vi "Insight_RW_Sweep_Power.vi"(7 "Parameter Type":enum16{"Value", "MAXimum", "MINimum", "DEFault"}(ring), 8 "error in (no error)":errorcluster, 9 "Mode (Read / Write)":enum8{"Write", "Read"}(ring), 10 "Power (mW)":dbl=5.0, 11 "telnet connection":T1) -> (0 "error out":errorcluster, 1 "response data":string, 2 "Power (mW)":dbl format="%.3g", 3 "telnet  connection out":T1)   [LabVIEW 2011]
doc: "Insight Photonic Solutions\n\nThis VI reads or writes the average power of the laser during a sweep.\n\nINPUTS\n\nMode - Tells the VI whether the command is a Read or a Write. (Default = Read).\nParameter Type - Tells the VI whether the command should use a Value or a keyword MAXimum, MINimum or DEFault to set the parameter value. (Default = Value).\nPower (mW) - The numeric value to set the average power of the laser during a sweep. (Default = 5).\nerror in - The standard LabView Error cluster. Use this to enforce sequentiality and error tracking.\n\nOUTPUTS\n\nresponse data - the complete response string from the laser\nPower (mW) - the average power written to or read from the laser\nerror out - the standard error cluster. Reports errors in reading or writing to the laser, or passes through errors from before this VI.\n\nver 1.0 - original release\nver 1.1 - returns the full response string and captures errors if parameter or command not recognized.\nver 3.2 - updated parser to accept responses from Atlas 3.1 and earlier or Atlas 3.2 and later.\nver 3.4 - added Insight CMD composer VI to enable setting values to MAX, MIN or DEFault."
uses:
  Telnet Session.ctl
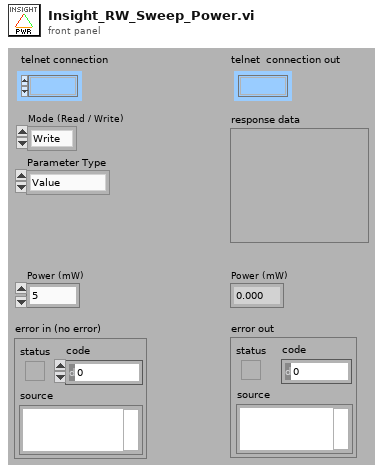
[diagram p1: front panel]
types:
  T1 = typedef "Telnet Session.ctl" = refnum<k1>
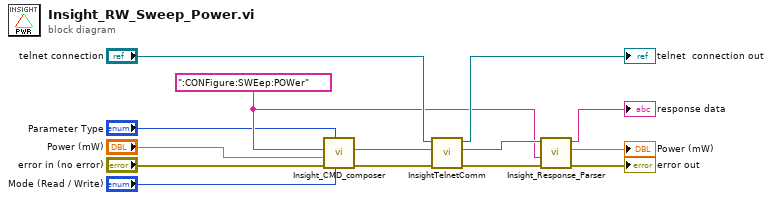
[diagram p0: block diagram]
diagram:
  w3 = ":CONFigure:SWEep:POWer" ("String")
  n1 = call "Insight_CMD_composer.vi"("Mode (Read / Write)"="Mode (Read / Write)", "Parameter Type"="Parameter Type", "error in (no error)"="error in (no error)", "Value"="Power (mW)", "CMD"=w3) -> ("error out"=w7:errorcluster, "Command String"=w5:string)  [unwired: 5 in]
  n2 = call "InsightTelnetComm.vi"("error in"=w7, "write buffer (\"\")"=w5, "telnet connection"="telnet connection") -> ("error out"=w12:errorcluster, "response data"=w8:string, "telnet  connection out"=→"telnet  connection out":T1)  [unwired: 4 in]
  n3 = call "Insight_Response_Parser.vi"("error in (no error)"=w12, "Command String"=w3, "Laser Response In"=w8) -> ("error out"=→"error out":errorcluster, "Value"=→"Power (mW)":dbl, "Laser Response Out"=→"response data":string)  [unwired: 6 in]
